vi "startup.vi"(8 "error in (no error)":errorcluster, 11 "PixelflySettings in":refnum<class "PixelflySettings.lvclass">) -> (0 "error out":errorcluster, 3 "PixelflySettings out":refnum<class "PixelflySettings.lvclass">)   [LabVIEW 2011, in "Tools.lvlib" / "Settings.lvlib" / "PixelflySettings.lvclass"]
uses:
  PixelflySettings.lvclass
  Filing/FileSystem/FileSystem.lvclass
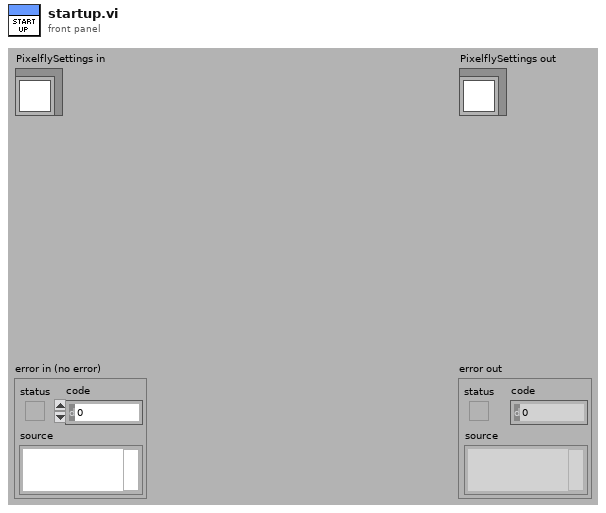
[diagram p1: front panel]
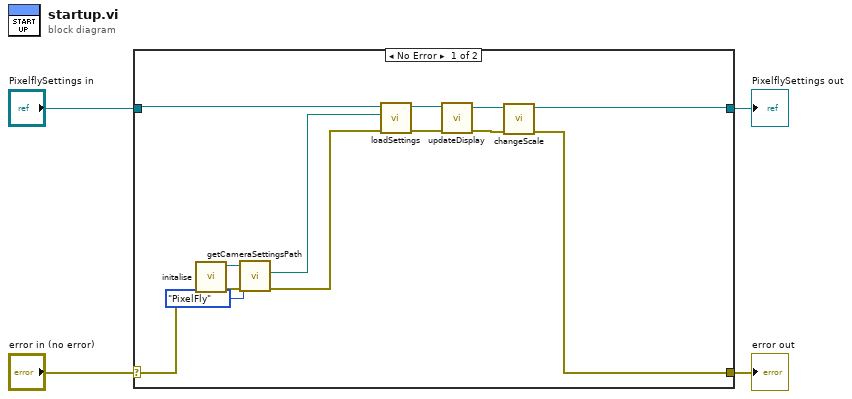
[diagram p0: block diagram]
diagram:
  n1 = case shown="No Error" "error in (no error)" {
    selector: "error in (no error)" -> [w11 w19]
    tunnel: [w6 w19] -> w3
    tunnel: [w7 w18] -> w1
    tunnel: "PixelflySettings in" -> [w17 w18]
    frame No Error {
      n2 = call "initalise.vi"("error in (no error)"=w11) -> ("error out"=w13:errorcluster, "FileSystem out"=w14:refnum<class "FileSystem.lvclass">)  [unwired: 9 in]
      n3 = call-dynamic "getCameraSettingsPath.vi"("error in (no error)"=w13, "Camera"=enum16{"Pixis", "ProEM", "PixelFly"}."PixelFly", "FileSystem.lvclass in"=w14) -> ("error out"=w10:errorcluster, "CameraSettingsPath"=w12:path)  [unwired: 6 in, 1 out]
      n4 = call-dynamic "loadSettings.vi"("error in (no error)"=w10, "Path"=w12, "PixelflySettings in"=w17) -> ("error out"=w15:errorcluster, "PixelflySettings out"=w16:refnum<class "PixelflySettings.lvclass">)  [unwired: 7 in]
      n5 = call "updateDisplay.vi"("error in (no error)"=w15, "PixelflySettings in"=w16) -> ("error out"=w8:errorcluster, "PixelflySettings out"=w9:refnum<class "PixelflySettings.lvclass">)  [unwired: 8 in]
      n6 = call "changeScale.vi"("error in (no error)"=w8, "PixelflySettings in"=w9) -> ("error out"=w6:errorcluster, "PixelflySettings out"=w7:refnum<class "PixelflySettings.lvclass">)  [unwired: 8 in]
    }
    frame Error {
    }
  }
  "error out" <- w3
  "PixelflySettings out" <- w1
